vi "Read age using variant.vi"(11 "variant in":variant) -> (1 "error out":errorcluster, 2 "age":dbl, 3 "variant out":variant)   [LabVIEW 2011]
uses:
  ClassDefinitions/SimpleClassWithProperties/myClass.lvclass
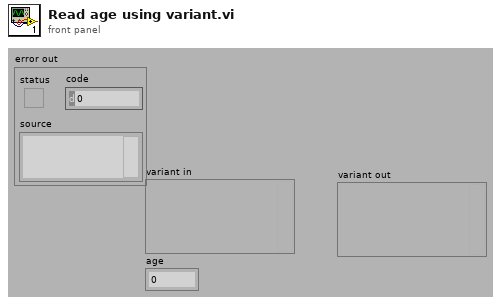
[diagram p1: front panel]
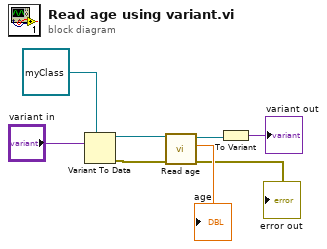
[diagram p0: block diagram]
diagram:
  n1 = Variant To Data(type=refnum<class "myClass.lvclass"> refnum ("myClass.lvclass"), Variant="variant in") -> (data=w5:refnum<class "myClass.lvclass">, error out=w6:errorcluster)  [unwired: 1 in]
  n2 = call-dynamic "Read age.vi"("error in (no error)"=w6, "myClass in"=w5) -> ("error out"=→"error out":errorcluster, "age"=→"age":dbl, "myClass out"=w4:refnum<class "myClass.lvclass">)  [unwired: 7 in]
  n3 = To Variant(anything=w4) -> (Variant=→"variant out":variant)
